vi "transistor curve.vi"() -> ()   [LabVIEW 2021]
uses:
  TransistorStateControl1.ctl
  <vilib>/Utility/file.llb/Write Delimited Spreadsheet (DBL).vi
panel:
  in  "EXIT":bool
  out "Num Graphs":dbl
  out "Boolean":bool
  in  "stop":bool
  out "XY Graph":cluster{dbl[], dbl[]}[](graph)
  in  "Collector Resistor":dbl
  in  "Base Resistor":dbl
  in  "Step Vcc (V)":dbl
  in  "Stop Vcc (V)":dbl
  in  "Start Vcc (V)":dbl
  in  "Step Current (uA)":dbl
  in  "Stop Current (uA)":dbl
  in  "Start Current (uA)":dbl
  in  "LOG":bool
  in  "run":bool
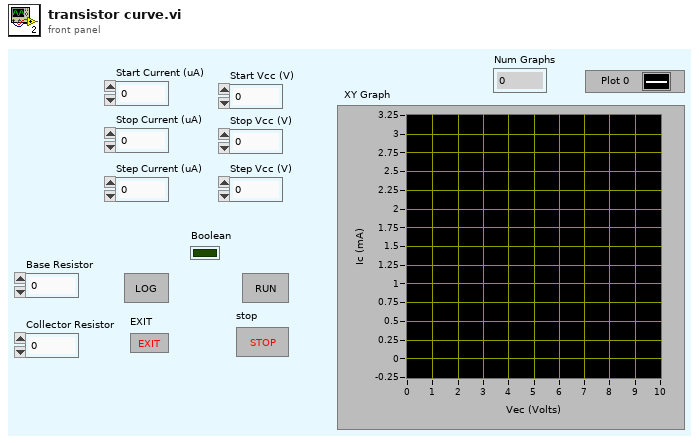
[diagram p1: front panel]
types:
  T1 = typedef "TransistorStateControl1.ctl" = enum16{"Initialization", "Wait for Command", "Run Test", "Save to Spreadsheet", "Exit"}
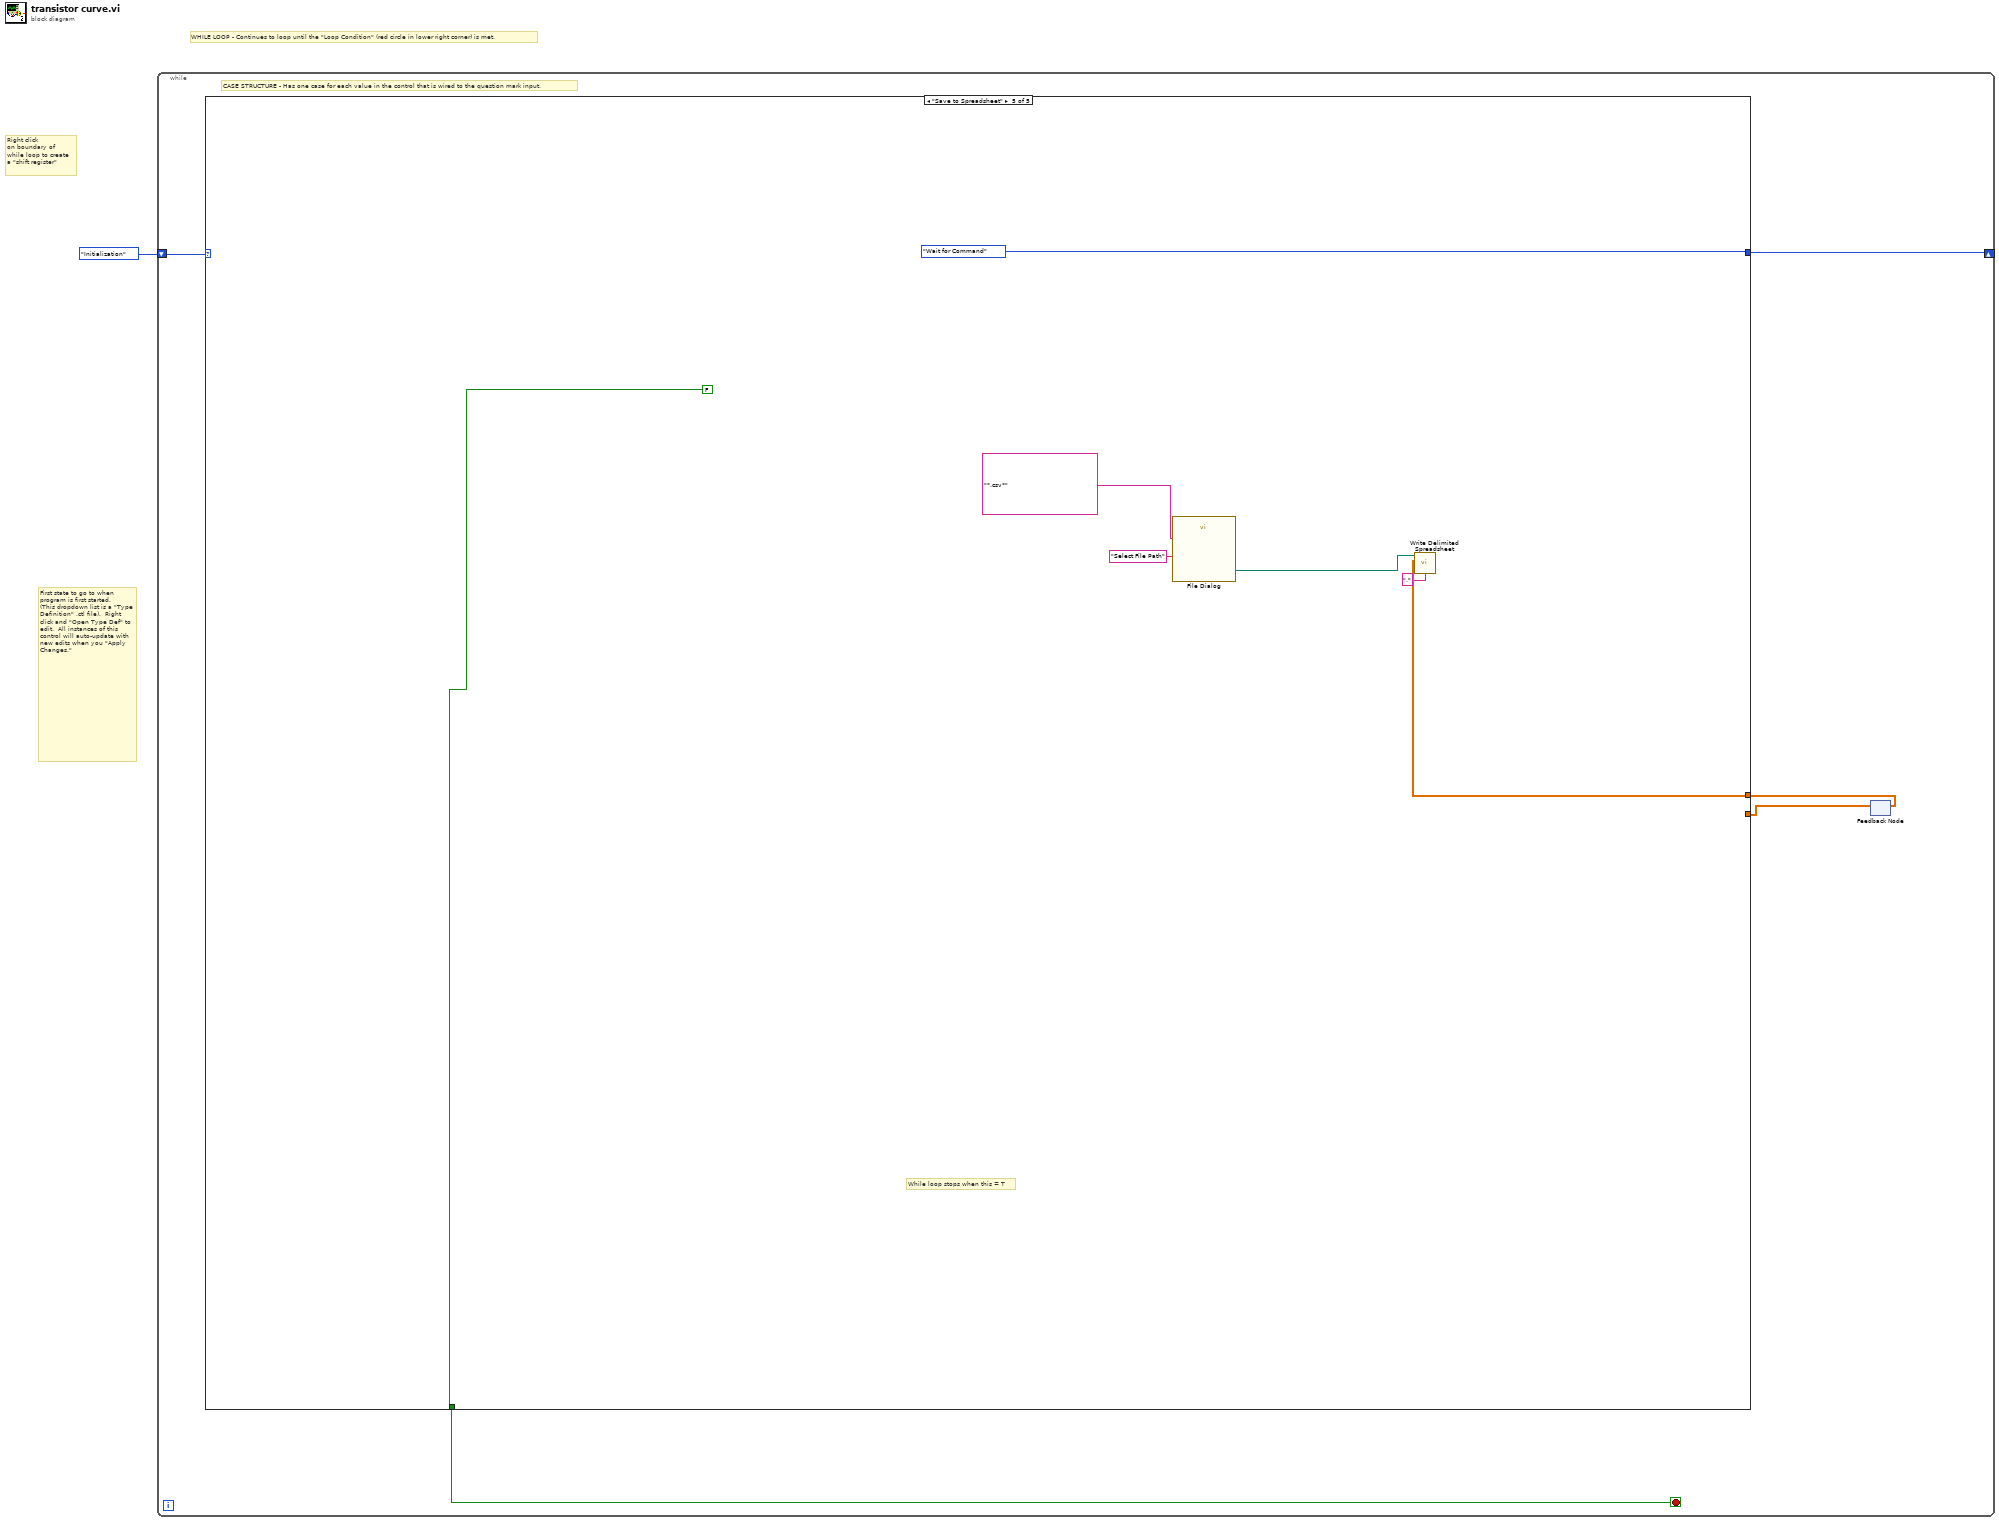
[diagram p0: block diagram]
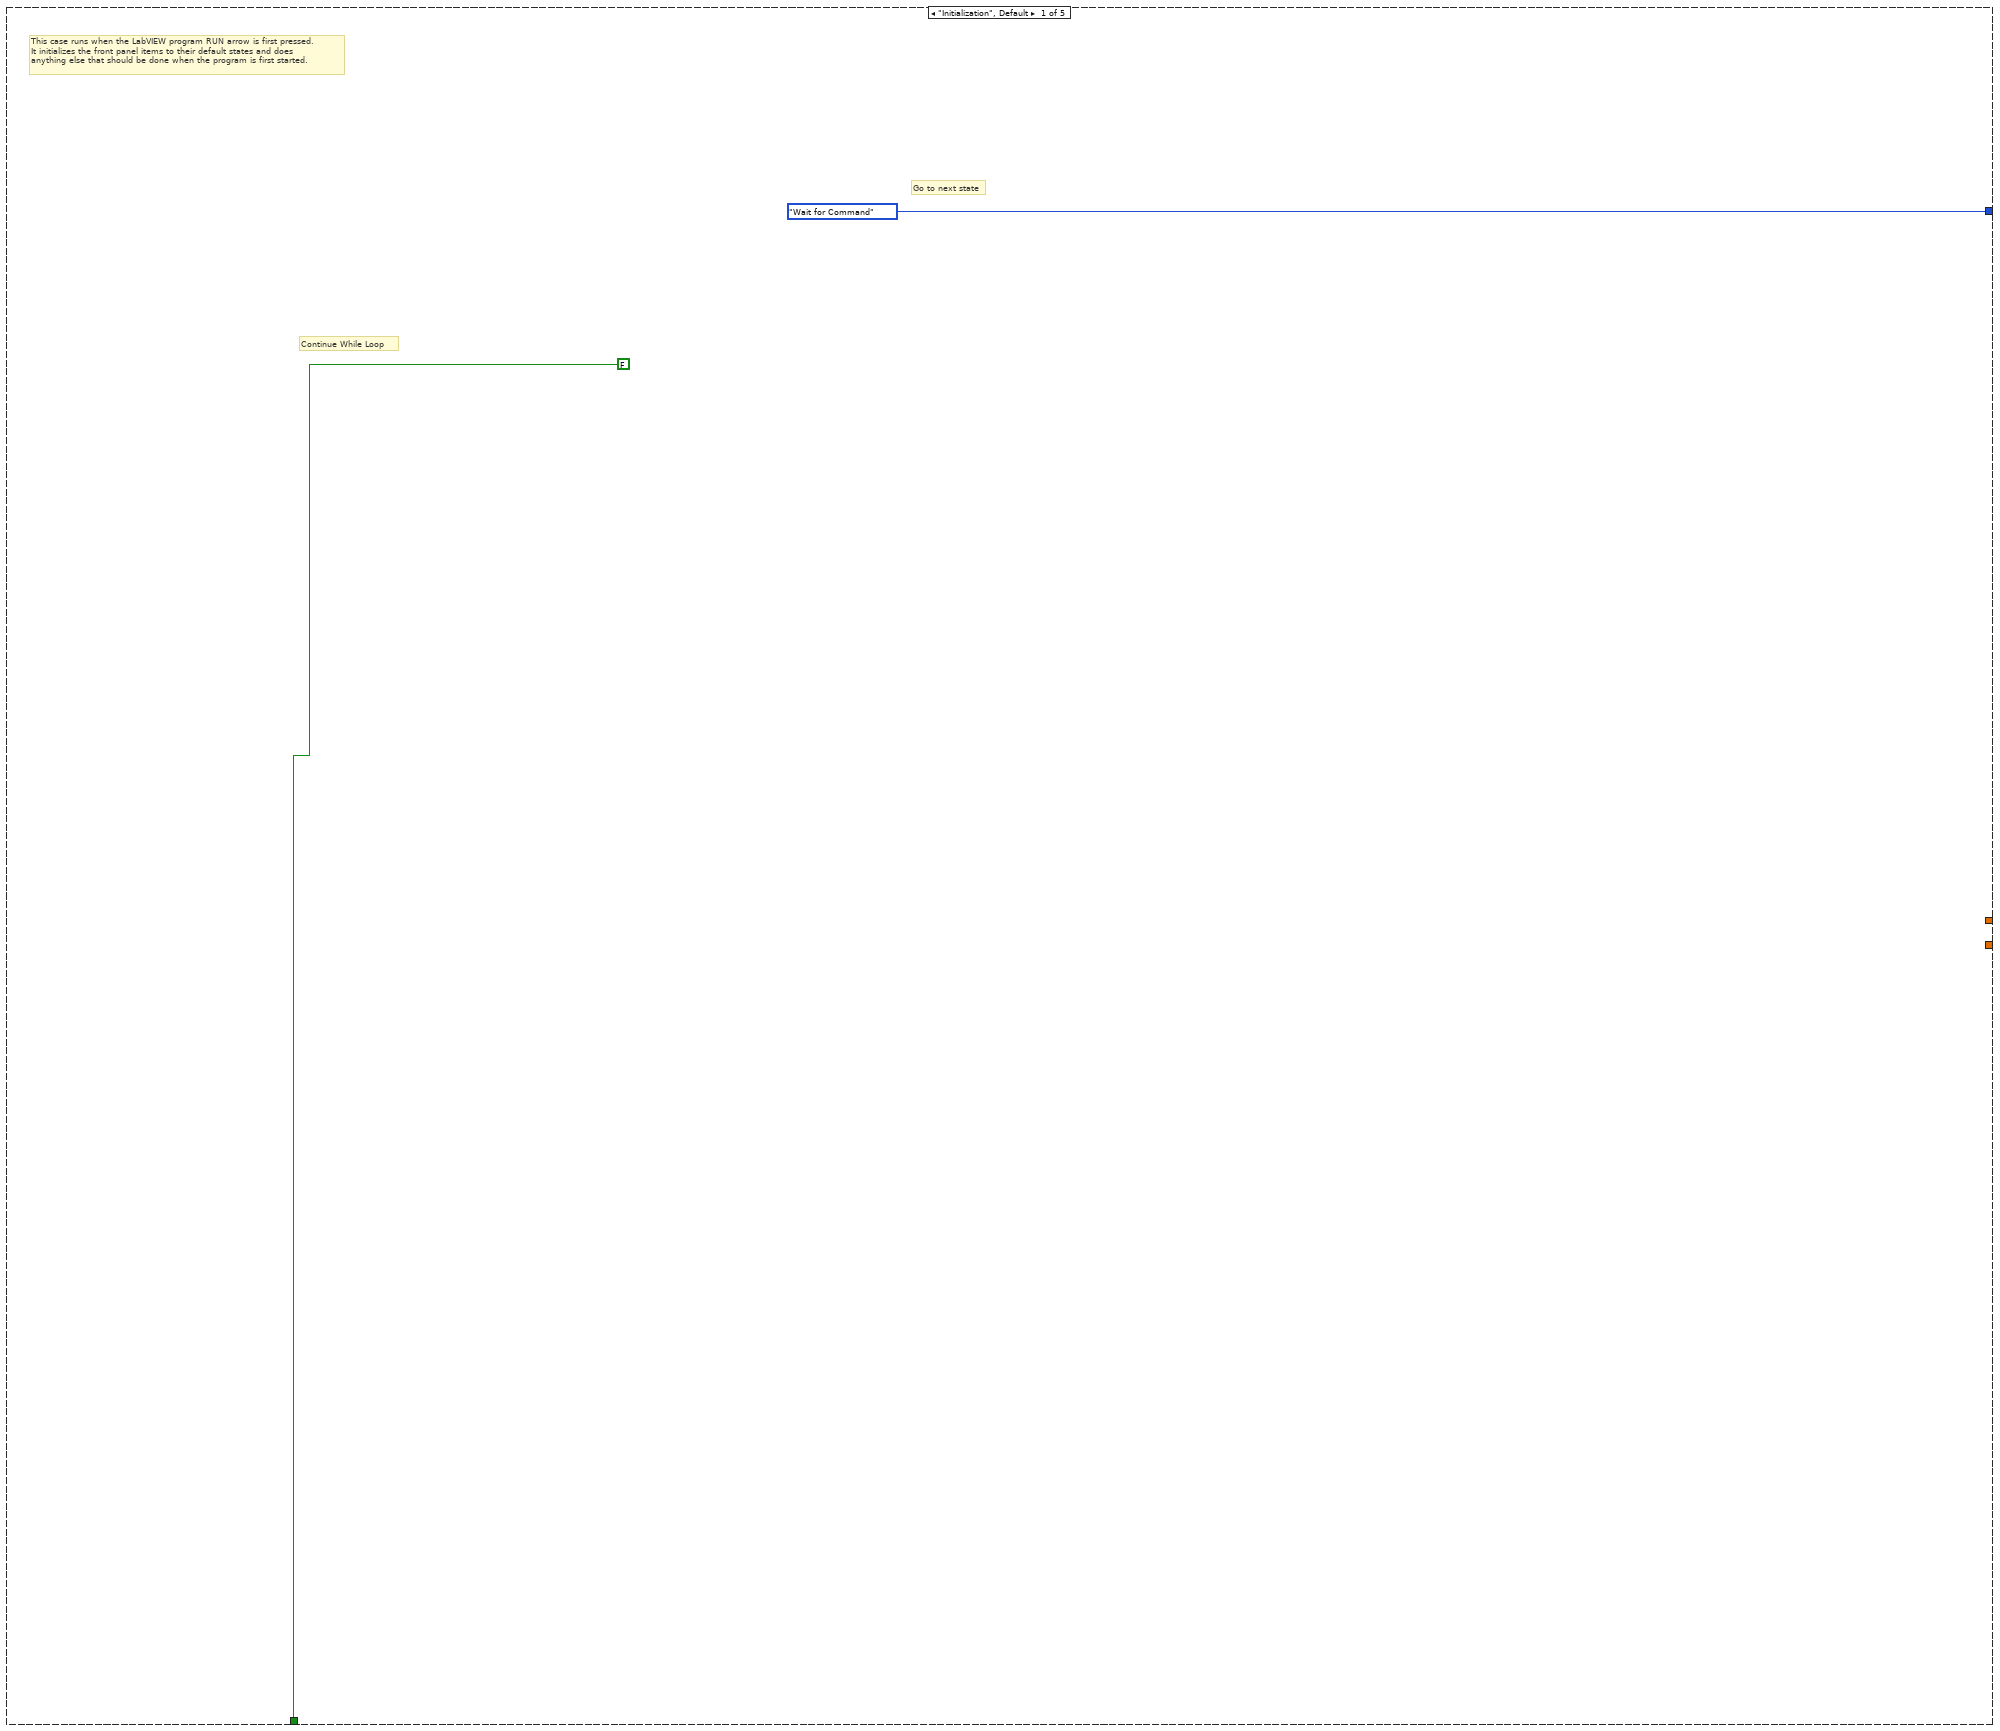
[diagram p2: hidden frame]
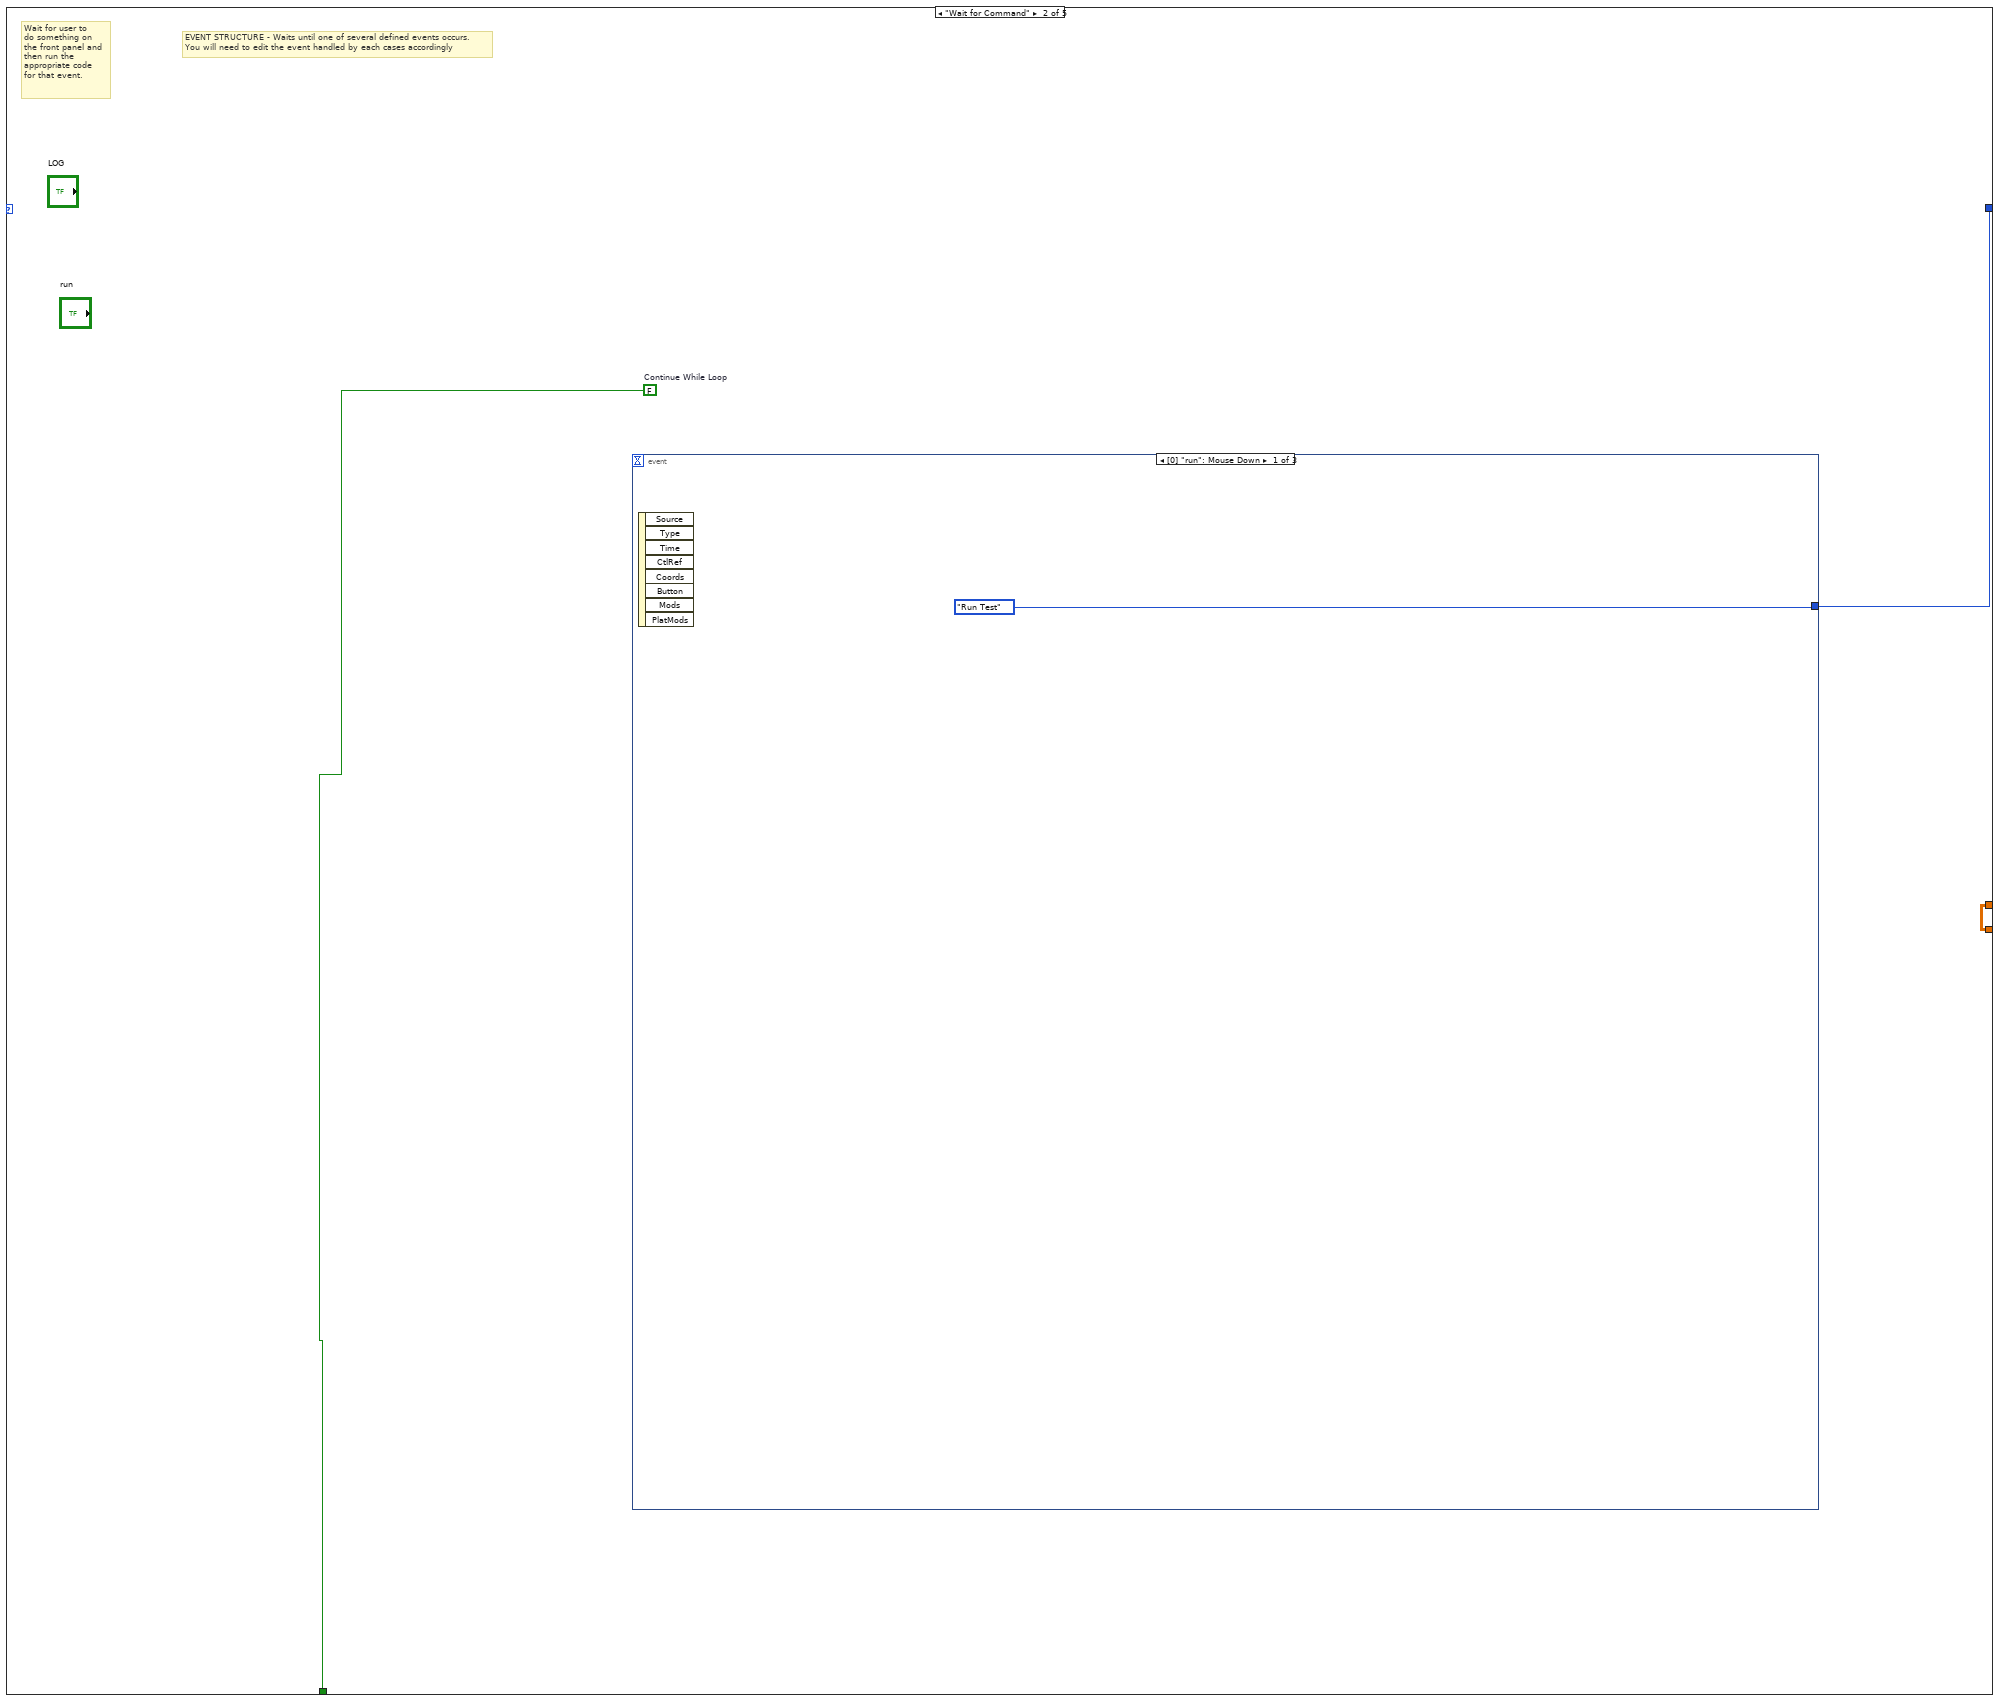
[diagram p3: hidden frame]
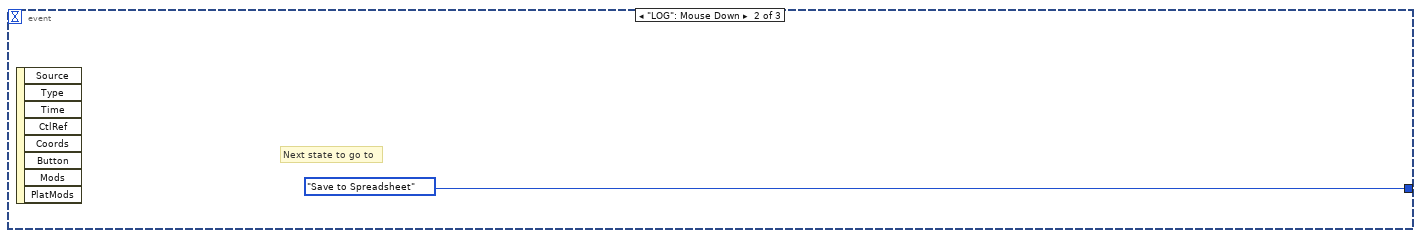
[diagram p4: hidden frame]
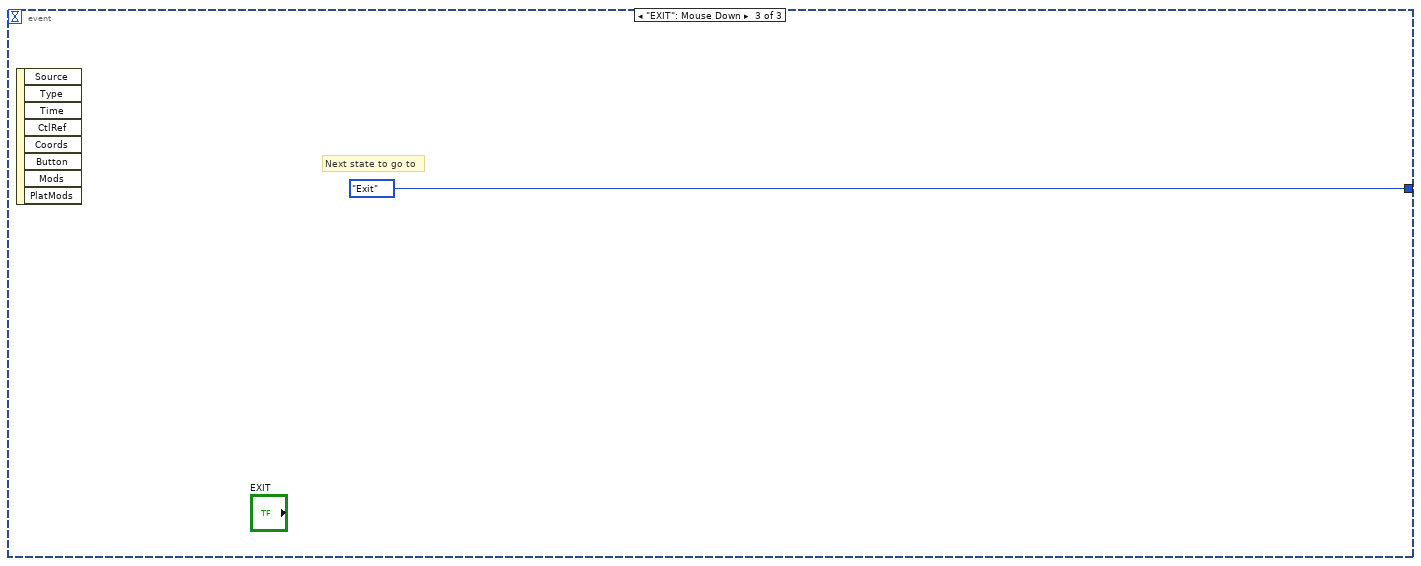
[diagram p5: hidden frame]
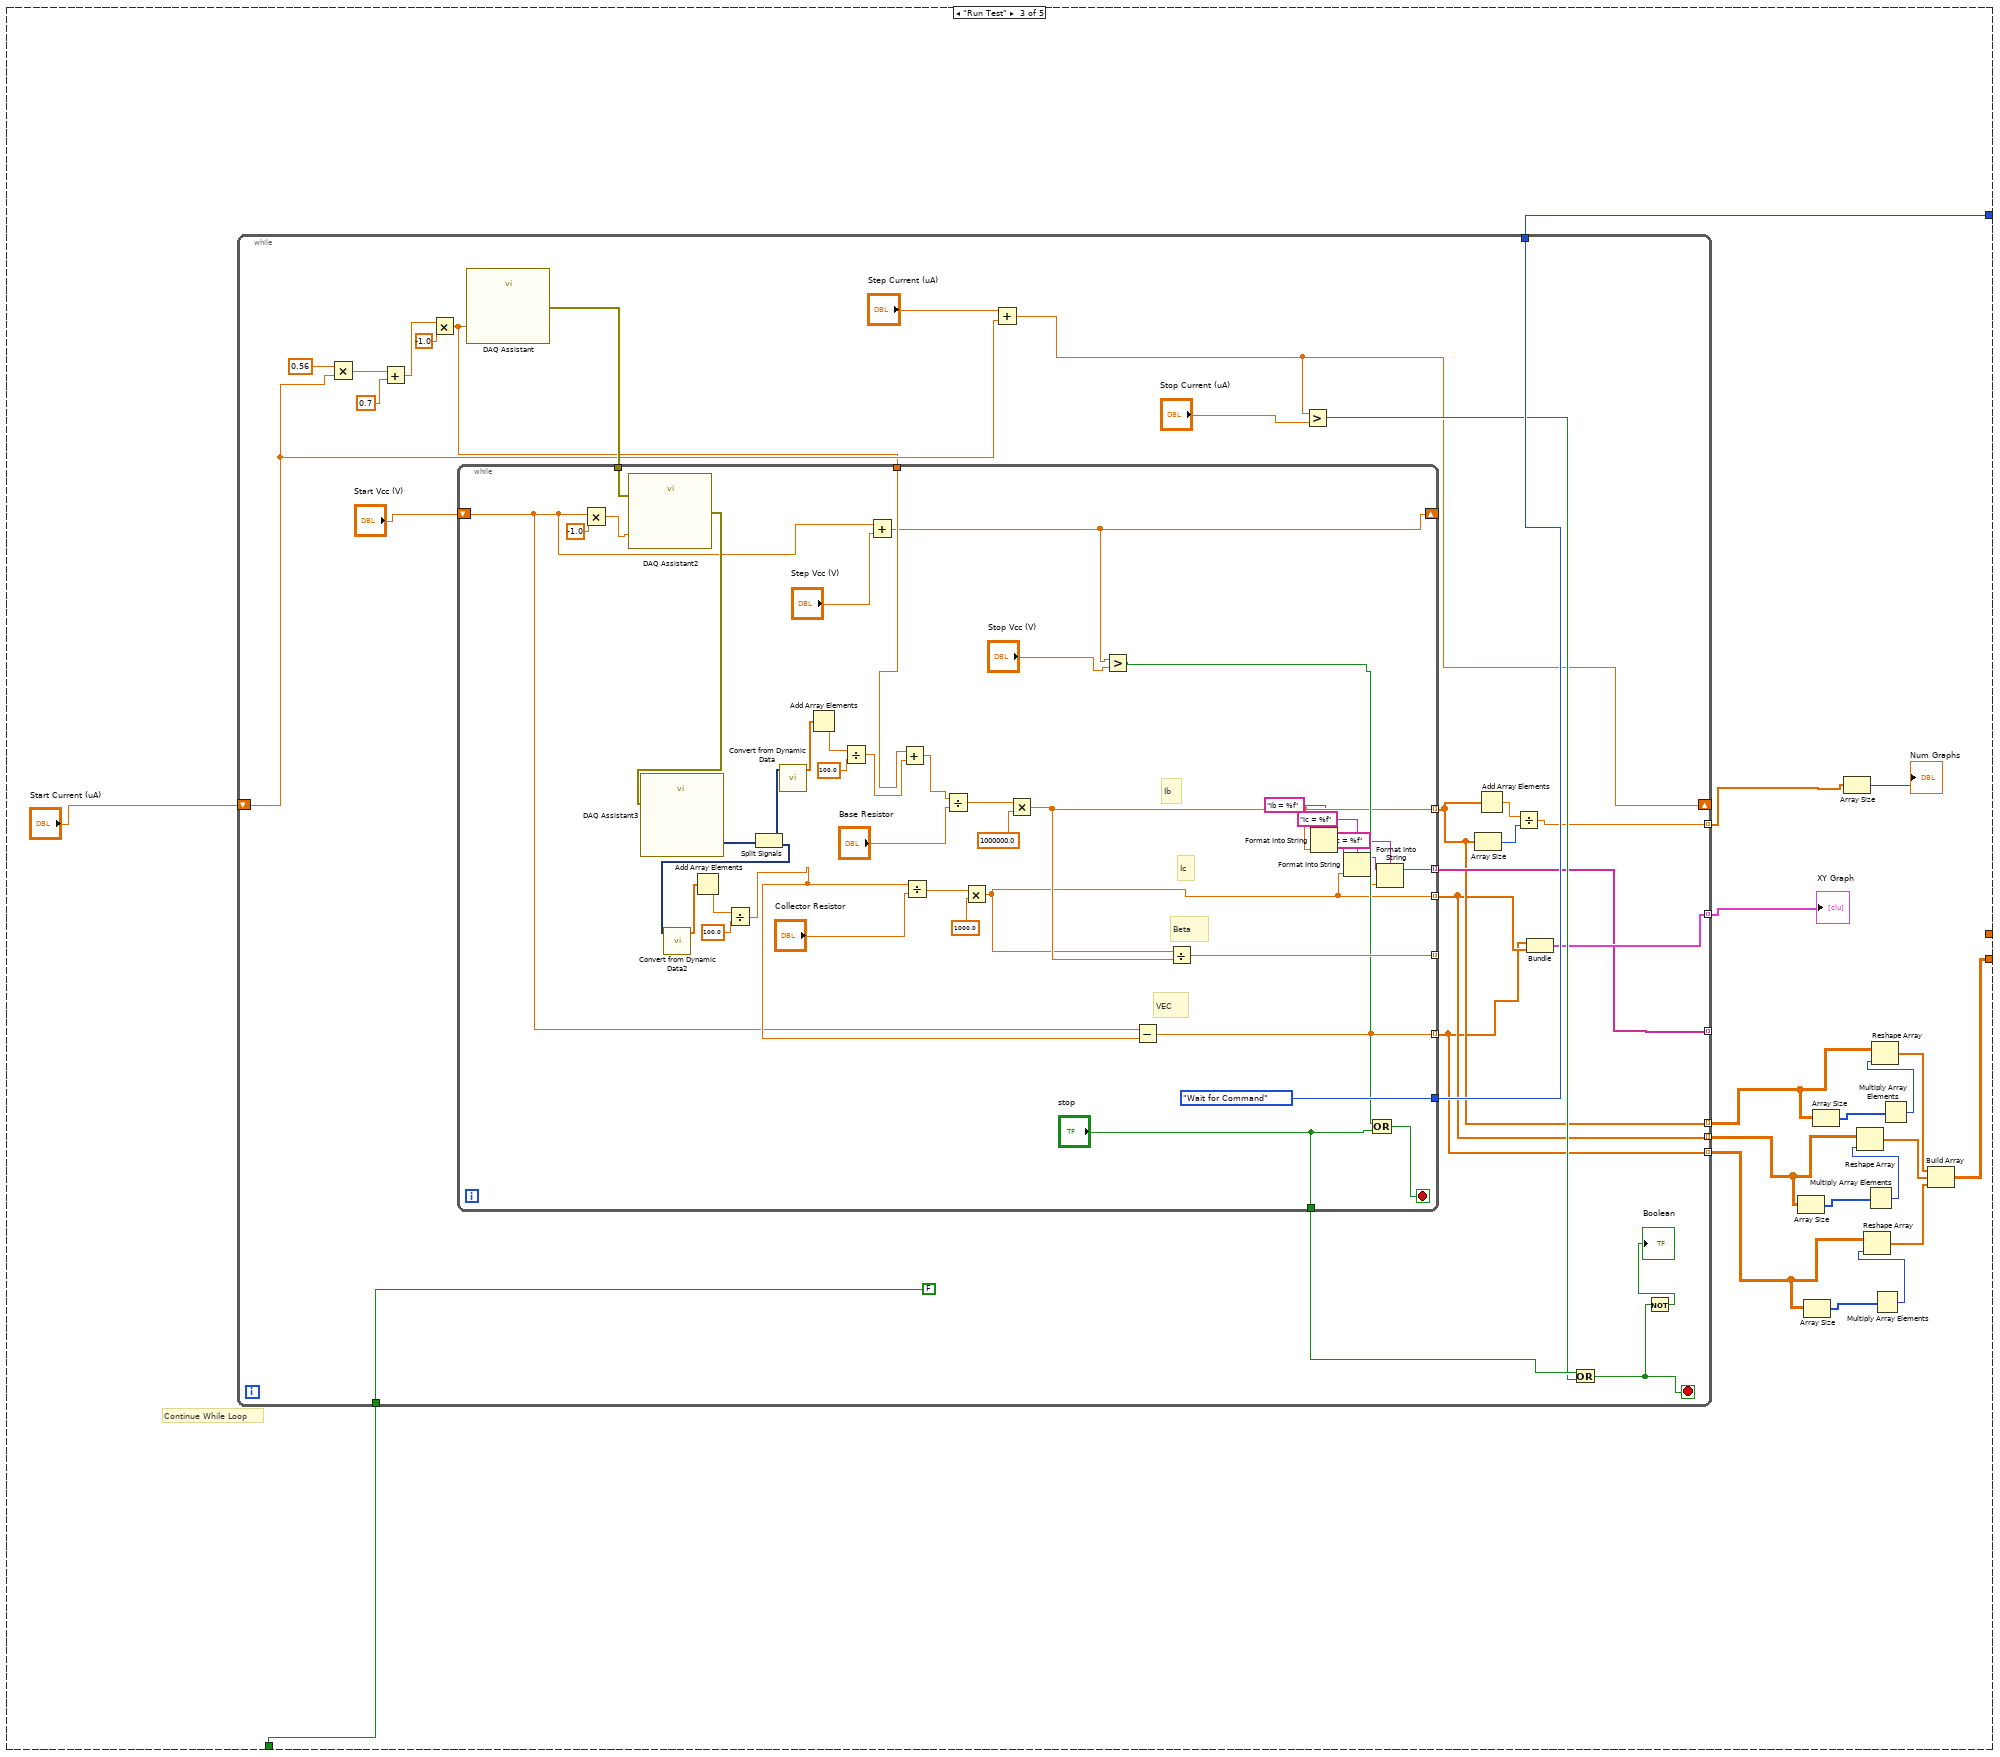
[diagram p6: hidden frame]
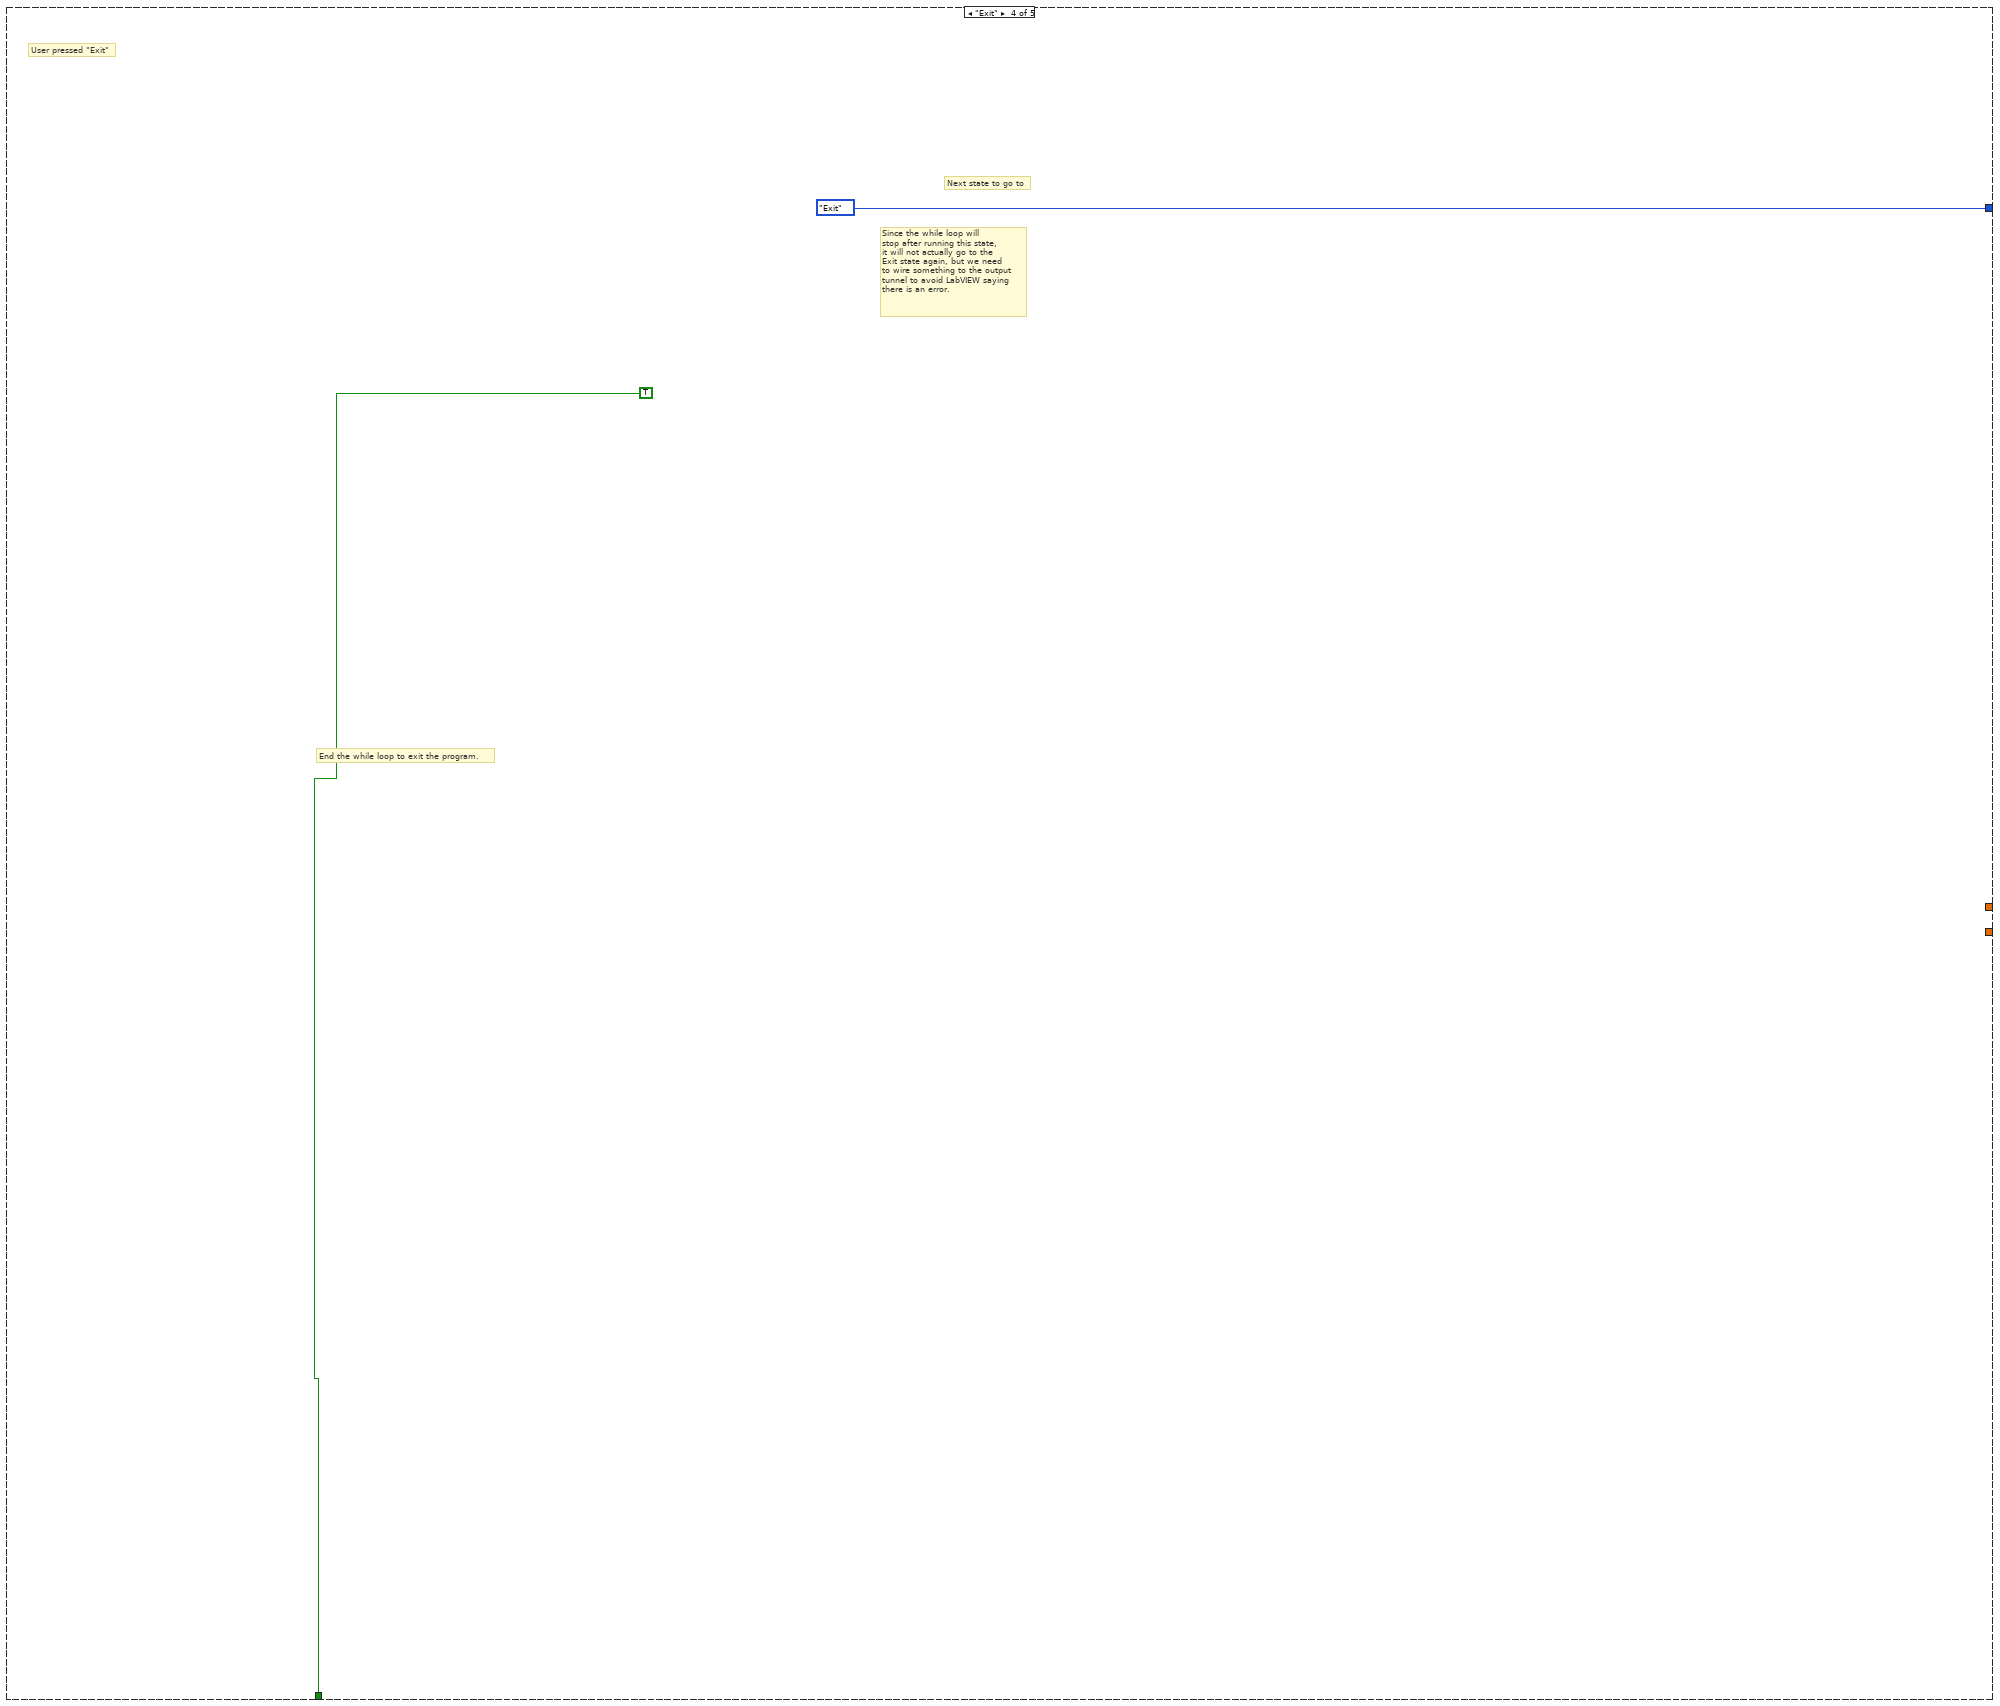
[diagram p7: hidden frame]
diagram:
  # "Right click\non boundary of\nwhile loop to create\na \"shift register\""
  # "WHILE LOOP - Continues to loop until the \"Loop Condition\" (red circle in lower right corner) is met."
  # "First state to go to when program is first started.\n(This dropdown list is a \"Type Definition\" .ctl file).  Right click and \"Open Type Def\" to edit.  All instances of this control will auto-update with new edits when you \"Apply Changes.\""
  n1 = while {
    shift-right: [w4] -> _
    shift-left: TransistorStateControl1."Initialization" ("Program State") -> [w5]
    stop <- w6 stop-if-true
    # "CASE STRUCTURE - Has one case for each value in the control that is wired to the question mark input."
    # "While loop stops when this = T"
    n2 = feedback #1() -> (w2:dbl[][])  [unwired: 1 in]
    n3 = case shown="\"Save to Spreadsheet\"" w5 {
      tunnel: [TransistorStateControl1."Wait for Command" ("Program State") w10 w33 TransistorStateControl1."Exit" ("Program State") TransistorStateControl1."Wait for Command" ("Program State")] -> w4
      tunnel: [FALSE w11 w32 TRUE FALSE] -> w6
      tunnel: [_ w9 w15 _ _] -> w3
      tunnel: w2 -> [_ w9 _ _ w105]
      frame "Initialization", Default {
        # "Continue While Loop"
        # "This case runs when the LabVIEW program RUN arrow is first pressed.\nIt initializes the front panel items to their default states and does\nanything else that should be done when the program is first started."
        # "Go to next state"
      }
      frame "Wait for Command" {
        w11 = FALSE  # Continue While Loop
        # "Wait for user to\ndo something on\nthe front panel and\nthen run the\nappropriate code\nfor that event."
        # "EVENT STRUCTURE - Waits until one of several defined events occurs.\nYou will need to edit the event handled by each cases accordingly"
        n4 = event shown="[0] \"run\": Mouse Down" {
          selector: _ -> [_ _ _]
          dyn-events: _ -> [_ _ _]
          timeout: _ -> [_ _ _]
          tunnel: [TransistorStateControl1."Run Test" ("Program State") TransistorStateControl1."Save to Spreadsheet" ("Program State") TransistorStateControl1."Exit" ("Program State")] -> w10
          event "run": Mouse Down {
            n5 = event-data() -> ()  [unwired: 1 in, 8 out]
          }
          event "LOG": Mouse Down {
            # "Next state to go to"
            n6 = event-data() -> ()  [unwired: 1 in, 8 out]
          }
          event "EXIT": Mouse Down {
            # "Next state to go to"
            n7 = event-data() -> ()  [unwired: 1 in, 8 out]
          }
        }
      }
      frame "Run Test" {
        # "Continue While Loop"
        n8 = while {
          tunnel: [w52] -> w33
          tunnel: [FALSE] -> w32
          shift-right: [w40] -> _
          shift-left: "Start Current (uA)" -> [w41]
          tunnel: [w38] -> w28 mode=indexing
          tunnel: [w44] -> w29 mode=indexing
          tunnel: [w37] -> _ mode=indexing
          tunnel: [w36] -> w25 mode=indexing
          tunnel: [w35] -> w20 mode=indexing
          tunnel: [w34] -> w19 mode=indexing
          stop <- w47 stop-if-true
          n9 = Multiply(x=0.56, y=w41) -> (x*y=w56:dbl)
          n10 = Add(x=w56, y=0.7) -> (x+y=w42:dbl)
          n11 = Multiply(x=w42, y=-1.0) -> (x*y=w39:dbl)
          n12 = call "DAQ Assistant"("data"=w39) -> ("error out"=w45:errorcluster)  [unwired: 17 in, 1 out]
          n13 = while {
            shift-right: [w71] -> _
            shift-left: "Start Vcc (V)" -> [w75]
            tunnel: [w64] -> w34 mode=indexing
            tunnel: [w65] -> w35 mode=indexing
            tunnel: [w66] -> w36 mode=indexing
            tunnel: [w93] -> _ mode=indexing
            tunnel: [TransistorStateControl1."Wait for Command" ("Program State")] -> w52
            tunnel: ["stop"] -> w51
            tunnel: w45 -> [w89]
            tunnel: w39 -> [w74]
            tunnel: [w60] -> w37 mode=indexing
            stop <- w92 stop-if-true
            # "VEC"
            # "Beta"
            # "Ic"
            # "Ib"
            n14 = Multiply(x=w75, y=-1.0) -> (x*y=w76:dbl)
            n15 = call "DAQ Assistant2"("data"=w76, "error in"=w89) -> ("error out"=w88:errorcluster)  [unwired: 16 in, 1 out]
            n16 = call "DAQ Assistant3"("error in"=w88) -> ("data"=w87:dynamicdata)  [unwired: 16 in, 2 out]
            n17 = Split Signals(w87) -> (w86:dynamicdata, w79:dynamicdata)  [unwired: 2 in]
            n18 = call "Convert from Dynamic Data2"("Dynamic Data Type"=w79) -> ("Array"=w82:dbl[])  [unwired: 3 in]
            n19 = Add Array Elements(numeric array=w82) -> (sum=w81:dbl)
            n20 = Divide(x=w81, y=100.0) -> (x/y=w78:dbl)
            n21 = call "Convert from Dynamic Data"("Dynamic Data Type"=w86) -> ("Array"=w85:dbl[])  [unwired: 3 in]
            n22 = Add Array Elements(numeric array=w85) -> (sum=w84:dbl)
            n23 = Divide(x=w84, y=100.0) -> (x/y=w73:dbl)
            n24 = Add(x=w75, y="Step Vcc (V)") -> (x+y=w71:dbl)
            n25 = Add(x=w74, y=w73) -> (x+y=w72:dbl)
            n26 = Divide(x=w78, y="Collector Resistor") -> (x/y=w94:dbl)
            n27 = Divide(x=w72, y="Base Resistor") -> (x/y=w97:dbl)
            n28 = Multiply(x=w94, y=1000.0) -> (x*y=w65:dbl)
            n29 = Multiply(x=w97, y=1000000.0) -> (x*y=w66:dbl)
            n30 = Greater?(x=w71, y="Stop Vcc (V)") -> (0:w69:bool)
            n31 = Subtract(x=w75, y=w78) -> (x-y=w64:dbl)
            n32 = Divide(x=w65, y=w66) -> (x/y=w93:dbl)
            n33 = Format Into String(format string="Ib = %f", w66) -> (resulting string=w68:string)  [unwired: 2 in, 1 out]
            n34 = Format Into String(format string="Ic = %f", initial string=w68, w65) -> (resulting string=w67:string)  [unwired: 1 in, 1 out]
            n35 = Or(x=w69, y="stop") -> (x .or. y?=w92:bool)
            n36 = Format Into String(format string="Vec = %f", initial string=w67, w64) -> (resulting string=w60:string)  [unwired: 1 in, 1 out]
          }
          n37 = Add(x="Step Current (uA)", y=w41) -> (x+y=w40:dbl)
          n38 = Greater?(x=w40, y="Stop Current (uA)") -> (0:w48:bool)
          n39 = Array Size(array=w36) -> (size(s)=w53:i32)
          n40 = Add Array Elements(numeric array=w36) -> (sum=w54:dbl)
          n41 = Divide(x=w54, y=w53) -> (x/y=w38:dbl)
          n42 = Bundle(w34, w35) -> (w44:cluster{dbl[], dbl[]})  [unwired: 1 in]
          n43 = Or(x=w51, y=w48) -> (x .or. y?=w47:bool)
          n44 = Not(x=w47) -> (.not. x?=→"Boolean":bool)
        }
        "XY Graph" <- w29
        n45 = Array Size(array=w20) -> (size(s)=w24:i32[])
        n46 = Array Size(array=w19) -> (size(s)=w22:i32[])
        n47 = Array Size(array=w25) -> (size(s)=w27:i32[])
        n48 = Array Size(array=w28) -> (size(s)=→"Num Graphs":i32)
        n49 = Multiply Array Elements(1:w24) -> (0:w23:i32)
        n50 = Reshape Array(w20, w23) -> (w17:dbl[])
        n51 = Multiply Array Elements(1:w22) -> (0:w21:i32)
        n52 = Reshape Array(w19, w21) -> (w16:dbl[])
        n53 = Multiply Array Elements(1:w27) -> (0:w26:i32)
        n54 = Reshape Array(w25, w26) -> (w18:dbl[])
        n55 = Build Array(w18, w17, w16) -> (w15:dbl[][])
      }
      frame "Exit" {
        # "User pressed \"Exit\""
        # "End the while loop to exit the program."
        # "Since the while loop will\nstop after running this state,\nit will not actually go to the \nExit state again, but we need\nto wire something to the output\ntunnel to avoid LabVIEW saying\nthere is an error."
        # "Next state to go to"
      }
      frame "Save to Spreadsheet" {
        n56 = call "File Dialog"("prompt"="Select File Path", "pattern (all files)"="*.csv*") -> ("selected path"=w104:path)  [unwired: 10 in, 3 out]
        n57 = call-poly <vilib>:"Write Delimited Spreadsheet.vi"("file path (dialog if empty)"=w104, "2D data"=w105, "delimiter (\\t)"="," ("delimiter (\\t)")) -> ()  [unwired: 11 in, 2 out]
      }
    }
    n58 = feedback-in #1(w3) -> ()
  }
